vi "append_data.vi"(8 "error in (no error)":errorcluster, 10 "Current measurement #":i32, 11 "Counter in":refnum<class "Counter.lvclass">) -> (0 "error out":errorcluster, 3 "Counter out":refnum<class "Counter.lvclass">)   [LabVIEW 2014, in "Counter.lvclass"]
uses:
  Counter.lvclass
  Counter.lvclass/Counter.ctl
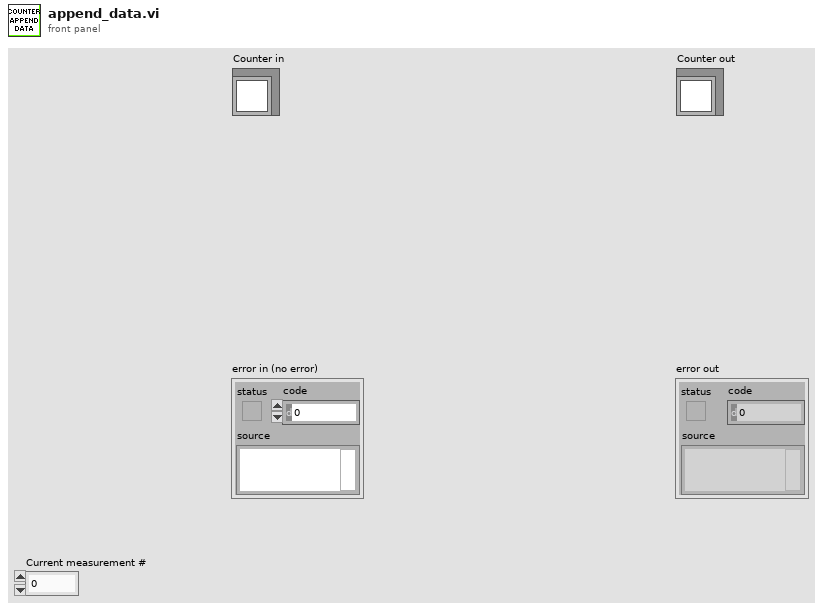
[diagram p1: front panel]
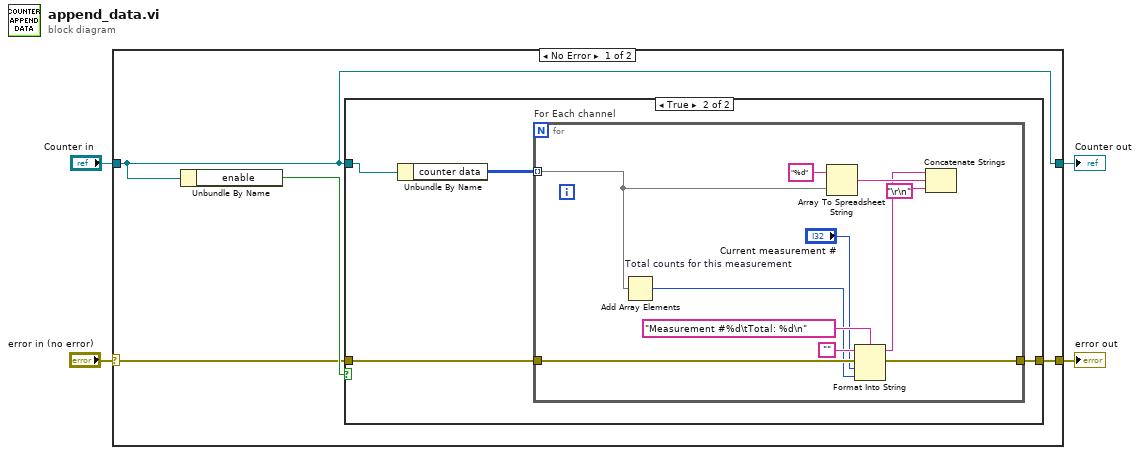
[diagram p0: block diagram]
diagram:
  n1 = case shown="No Error" "error in (no error)" {
    selector: "error in (no error)" -> [w7 w26]
    tunnel: [w5 w25] -> w2
    tunnel: "Counter in" -> [w5 w25]
    tunnel: [w6 w26] -> w1
    frame No Error {
      n2 = Unbundle By Name(w5) -> ("enable"=w8:bool)
      n3 = case shown="True" w8 {
        tunnel: w7 -> [w9 w13]
        tunnel: [w9 w12] -> w6
        tunnel: w5 -> [_ w11]
        frame False {
        }
        frame True {
          n4 = Unbundle By Name(w11) -> ("counter data"=w10:u32[][])
          n5 = for "For Each channel" {
            tunnel: w13 -> [w24]
            tunnel: [w15] -> w12
            tunnel: w10 -> [w14] mode=indexing
            n6 = Add Array Elements "Total counts for this measurement"(numeric array=w14) -> (sum=w17:u32)
            n7 = Array To Spreadsheet String(array=w14, 3:"%d" ("format string")) -> (spreadsheet string=w20:string)  [unwired: 1 in]
            n8 = Format Into String(format string="Measurement #%d\tTotal: %d\n", initial string="", error in=w24, "Current measurement #", w17) -> (resulting string=w19:string, error out=w15:errorcluster)
            n9 = Concatenate Strings(w19, w20, "\r\n") -> ()  [unwired: 1 out]
          }
        }
      }
    }
    frame Error {
    }
  }
  "error out" <- w1
  "Counter out" <- w2
